vi "AutoManipulator.vi"(8 "Time":u32, 11 "array":dbl[][](array[numeric])) -> ()   [LabVIEW 2019]
uses:
  <vilib>/Rock Robotics/WPI/ThirdParty/Phoenix-LabVIEW/Motor Controller/Controls/CTRE_Phoenix_MotorControl_ControlMode.ctl
  <vilib>/Rock Robotics/WPI/Solenoid/WPI_SolenoidValue.ctl
  6d52bef7-996c-4b1c-a658-80540290107b.vi
  <vilib>/Rock Robotics/WPI/Solenoid/WPI_SolenoidSetEnum.vi
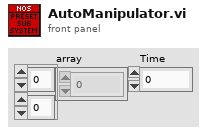
[diagram p1: front panel]
types:
  T1 = enum16{"Reserve", "Intake On", "Shooter On", "Shooter Spin Up"}
  T2 = typedef "WPI_MotorControlDeviceRef.ctl" = cluster{"DeviceStatus":errorcluster, "Type":T3, "PWM":cluster{"PWM Channel":T4, "DeadBand":T5}, "CAN":cluster{"Device Number":u8, "SetOutput VI Ref":variant, "GetOutput VI Ref":variant, "Enable VI Ref":variant, "Disable VI Ref":variant, "Data":variant}, "Invert":bool, "DIO PWM":cluster{"PWM \"Enable\" Channel":T4, "DIOChannel":T6, "PWM Rate":dbl}}
  T3 = typedef "WPI_MotorControlType.ctl" = enum16{"PWM", "CAN", "DIO PWM"}
  T4 = typedef "FPGA_DIOPWMChannel.ctl" = enum8{"PWM 0", "PWM 1", "PWM 2", "PWM 3", "PWM 4", "PWM 5", "PWM 6", "PWM 7", "PWM 8", "PWM 9", "PWM MXP 0", "PWM MXP 1", "PWM MXP 2", "PWM MXP 3", "PWM MXP 4", "PWM MXP 5", "PWM MXP 6", "PWM MXP 7", "PWM MXP 8", "PWM MXP 9", "Invalid"}
  T5 = typedef "WPI_PWMDeadband.ctl" = cluster{"Name":string, "maxPositivePwm":i32, "minPositivePwm":i32, "centerPwm":i32, "maxNegativePwm":i32, "minNegativePwm":i32, "angularRange":u16}
  T6 = typedef "FPGA_DIOChannel.ctl" = enum8{"DIO 0", "DIO 1", "DIO 2", "DIO 3", "DIO 4", "DIO 5", "DIO 6", "DIO 7", "DIO 8", "DIO 9", "DIO MXP 0", "DIO MXP 1", "DIO MXP 2", "DIO MXP 3", "DIO MXP 4", "DIO MXP 5", "DIO MXP 6", "DIO MXP 7", "DIO MXP 8", "DIO MXP 9", "DIO MXP 10", "DIO MXP 11", "DIO MXP 12", "DIO MXP 13", "DIO MXP 14", "DIO MXP 15", "SPI Port CS1", "SPI Port CS2", "SPI Port CS3", "SPI Port MISO", "SPI Port MOSI", "Invalid"}
  T7 = typedef "WPI_SolenoidDevRef.ctl" = cluster{"DevStatus":errorcluster, "Pneumatics Control Module":u8, "Forward Solenoid Channel":T8, "Reverse Solenoid Channel":T8}
  T8 = typedef "WPI_SolenoidChannel.ctl" = enum8{"Solenoid 0", "Solenoid 1", "Solenoid 2", "Solenoid 3", "Solenoid 4", "Solenoid 5", "Solenoid 6", "Solenoid 7", "Invalid"}
  T9 = typedef "WPI_SolenoidValue.ctl" = enum16{"Off", "On", "Forward", "Reverse"}
  T10 = typedef "CTRE_Phoenix_MotorControl_ControlMode.ctl" = u16
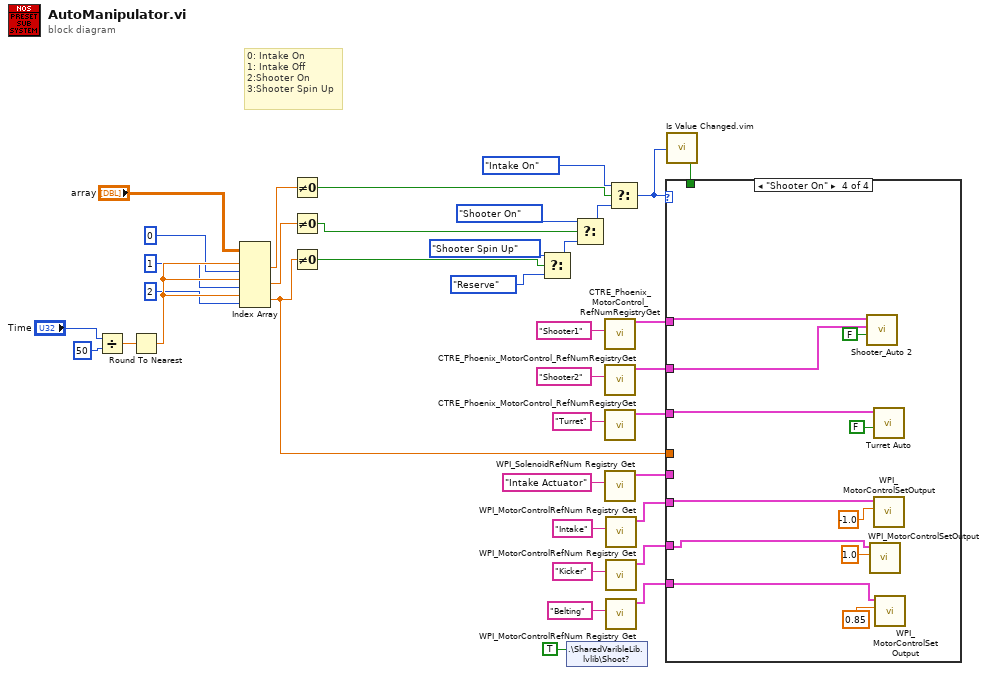
[diagram p0: block diagram]
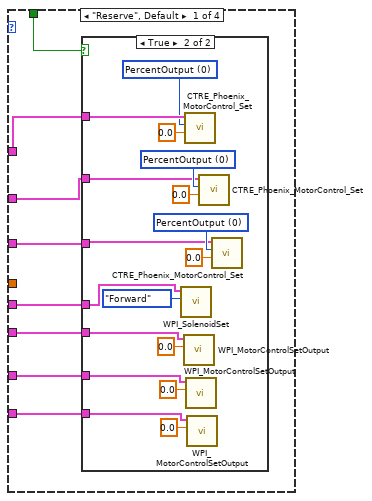
[diagram p2: hidden frame]
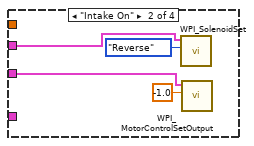
[diagram p4: hidden frame]
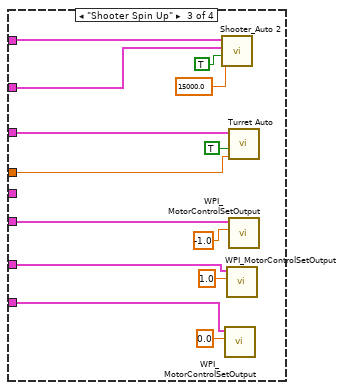
[diagram p5: hidden frame]
diagram:
  # "0: Intake On\n1: Intake Off\n2:Shooter On\n3:Shooter Spin Up"
  n1 = Divide(x="Time", y=u32 50) -> (x/y=w37:dbl)
  n2 = Round To Nearest(number=w37) -> (nearest integer value=w33:dbl)
  n3 = Index Array(array="array", index (row) #1=w33, index (col) #1=0 ("disabled index (col)"), index (row) #2=w33, index (col) #2=1 ("disabled index (col)"), index (row) #3=w33, index (col) #3=2 ("disabled index (col)")) -> (element #1=w32:dbl, element #2=w31:dbl, element #3=w7:dbl)
  n4 = Not Equal To 0?(x=w32) -> (x != 0?=w19:bool)
  n5 = Not Equal To 0?(x=w31) -> (x != 0?=w18:bool)
  n6 = Not Equal To 0?(x=w7) -> (x != 0?=w17:bool)
  n7 = Select(t=T1."Shooter Spin Up", s=w17, f=T1."Reserve") -> (s? t:f=w16:T1)
  n8 = shared-variable ".\\SharedVaribleLib.lvlib\\Shoot?"(TRUE ("Shoot?")) -> ()  [unwired: 1 in, 1 out]
  n9 = Select(t=T1."Shooter On", s=w18, f=w16) -> (s? t:f=w15:T1)
  n10 = call <vilib>:"CTRE_Phoenix_MotorControl_RefNumRegistryGet.vi"("refnum name"="Shooter1") -> ("PhoenixMotorControlDevRef"=w14:T2)  [unwired: 9 in, 1 out]
  n11 = call <vilib>:"CTRE_Phoenix_MotorControl_RefNumRegistryGet.vi"("refnum name"="Shooter2") -> ("PhoenixMotorControlDevRef"=w13:T2)  [unwired: 9 in, 1 out]
  n12 = call <vilib>:"CTRE_Phoenix_MotorControl_RefNumRegistryGet.vi"("refnum name"="Turret") -> ("PhoenixMotorControlDevRef"=w12:T2)  [unwired: 9 in, 1 out]
  n13 = call <vilib>:"WPI_SolenoidRefNum Registry Get.vi"("refnum name"="Intake Actuator") -> ("SolenoidDevRef"=w8:T7)  [unwired: 9 in, 1 out]
  n14 = call <vilib>:"WPI_MotorControlRefNum Registry Get.vi"("refnum name"="Intake") -> ("MotorControlDevRef"=w9:T2)  [unwired: 9 in, 1 out]
  n15 = call <vilib>:"WPI_MotorControlRefNum Registry Get.vi"("refnum name"="Kicker") -> ("MotorControlDevRef"=w10:T2)  [unwired: 9 in, 1 out]
  n16 = call <vilib>:"WPI_MotorControlRefNum Registry Get.vi"("refnum name"="Belting") -> ("MotorControlDevRef"=w11:T2)  [unwired: 9 in, 1 out]
  n17 = Select(t=T1."Intake On", s=w19, f=w15) -> (s? t:f=w2:T1)
  n18 = call "Is Value Changed.vim"("value"=w2) -> ("changed or first call?"=w1:bool)
  n19 = case shown="\"Shooter On\"" w2 {
    tunnel: w7 -> [_ _ w71 _]
    tunnel: w14 -> [w45 _ w79 w89]
    tunnel: w13 -> [w44 _ w78 w88]
    tunnel: w12 -> [w43 _ w76 w87]
    tunnel: w11 -> [w42 _ w67 w82]
    tunnel: w10 -> [w41 _ w69 w84]
    tunnel: w9 -> [w40 w63 w74 w86]
    tunnel: w8 -> [w39 w64 _ _]
    tunnel: w1 -> [w38 _ _ _]
    frame "Reserve", Default {
      n20 = case shown="True" w38 {
        tunnel: w45 -> [_ w62]
        tunnel: w44 -> [_ w57]
        tunnel: w43 -> [_ w54]
        tunnel: w42 -> [_ w50]
        tunnel: w41 -> [_ w49]
        tunnel: w40 -> [_ w48]
        tunnel: w39 -> [_ w46]
        frame False {
        }
        frame True {
          w56 = T10 0 items=["PercentOutput"=0, "Position"=1, "Velocity"=2, "Current"=3, "Follower"=5, "MotionProfile"=6, "MotionMagic"=7, "MotionProfileArc"=10, "Disabled"=15] ("Control Mode")
          w59 = T10 0 items=["PercentOutput"=0, "Position"=1, "Velocity"=2, "Current"=3, "Follower"=5, "MotionProfile"=6, "MotionMagic"=7, "MotionProfileArc"=10, "Disabled"=15] ("Control Mode")
          w61 = T10 0 items=["PercentOutput"=0, "Position"=1, "Velocity"=2, "Current"=3, "Follower"=5, "MotionProfile"=6, "MotionMagic"=7, "MotionProfileArc"=10, "Disabled"=15] ("Control Mode")
          n21 = call-poly <vilib>:"WPI_SolenoidSet.vi"("Value"=WPI_SolenoidValue."Forward", "SolenoidDevRef"=w46) -> ()  [unwired: 8 in, 2 out]
          n22 = call <vilib>:"WPI_MotorControlSetOutput.vi"("Output"=0.0, "MotorControlDevRef"=w48) -> ()  [unwired: 7 in, 3 out]
          n23 = call <vilib>:"CTRE_Phoenix_MotorControl_Set.vi"("Output"=0.0, "Control Mode"=w61, "PhoenixMotorControlDevRef"=w62) -> ()  [unwired: 7 in, 2 out]
          n24 = call <vilib>:"WPI_MotorControlSetOutput.vi"("Output"=0.0, "MotorControlDevRef"=w49) -> ()  [unwired: 7 in, 3 out]
          n25 = call <vilib>:"WPI_MotorControlSetOutput.vi"("Output"=0.0, "MotorControlDevRef"=w50) -> ()  [unwired: 7 in, 3 out]
          n26 = call <vilib>:"CTRE_Phoenix_MotorControl_Set.vi"("Output"=0.0, "Control Mode"=w59, "PhoenixMotorControlDevRef"=w57) -> ()  [unwired: 7 in, 2 out]
          n27 = call <vilib>:"CTRE_Phoenix_MotorControl_Set.vi"("Output"=0.0, "Control Mode"=w56, "PhoenixMotorControlDevRef"=w54) -> ()  [unwired: 7 in, 2 out]
        }
      }
    }
    frame "Intake On" {
      n28 = call-poly <vilib>:"WPI_SolenoidSet.vi"("Value"=WPI_SolenoidValue."Reverse", "SolenoidDevRef"=w64) -> ()  [unwired: 8 in, 2 out]
      n29 = call <vilib>:"WPI_MotorControlSetOutput.vi"("Output"=-1.0, "MotorControlDevRef"=w63) -> ()  [unwired: 7 in, 3 out]
    }
    frame "Shooter Spin Up" {
      n30 = call "Shooter_Auto 2.vi"("RPM Override"=15000.0, "Override?"=TRUE, "Followers"=w78, "Master"=w79) -> ()  [unwired: 8 in]
      n31 = call <vilib>:"WPI_MotorControlSetOutput.vi"("Output"=0.0, "MotorControlDevRef"=w67) -> ()  [unwired: 7 in, 3 out]
      n32 = call <vilib>:"WPI_MotorControlSetOutput.vi"("Output"=1.0, "MotorControlDevRef"=w69) -> ()  [unwired: 7 in, 3 out]
      n33 = call "Turret Auto.vi"("Override_Value"=w71, "Overide"=TRUE, "Motor1Ref"=w76) -> ()  [unwired: 9 in]
      n34 = call <vilib>:"WPI_MotorControlSetOutput.vi"("Output"=-1.0, "MotorControlDevRef"=w74) -> ()  [unwired: 7 in, 3 out]
    }
    frame "Shooter On" {
      n35 = call "Shooter_Auto 2.vi"("Override?"=FALSE, "Followers"=w88, "Master"=w89) -> ()  [unwired: 9 in]
      n36 = call <vilib>:"WPI_MotorControlSetOutput.vi"("Output"=1.0, "MotorControlDevRef"=w84) -> ()  [unwired: 7 in, 3 out]
      n37 = call "Turret Auto.vi"("Overide"=FALSE, "Motor1Ref"=w87) -> ()  [unwired: 10 in]
      n38 = call <vilib>:"WPI_MotorControlSetOutput.vi"("Output"=-1.0, "MotorControlDevRef"=w86) -> ()  [unwired: 7 in, 3 out]
      n39 = call <vilib>:"WPI_MotorControlSetOutput.vi"("Output"=0.85, "MotorControlDevRef"=w82) -> ()  [unwired: 7 in, 3 out]
    }
  }
